vi "Msg.vi"(7 "Actor in":refnum<class "Actor.lvclass">, 11 "Stop Msg in":refnum<class "Stop Msg.lvclass">) -> (0 "Error out":errorcluster, 5 "Actor out":refnum<class "Actor.lvclass">)   [LabVIEW 2025, in "jettl.lvlib" / "Stop Msg.lvlib" / "Stop Msg.lvclass"]
uses:
  Stop Msg.lvclass
  Actor/Actor/Actor.lvclass
  Stop/Stop.lvclass
  Stop Msg.lvclass/Stop Msg.ctl
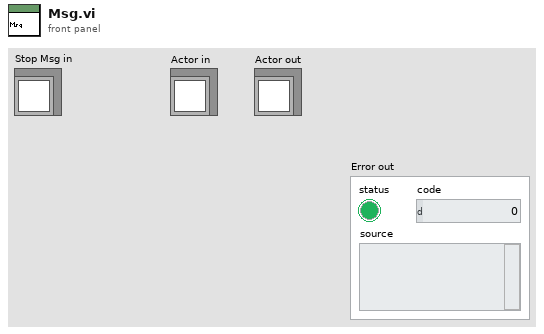
[diagram p1: front panel]
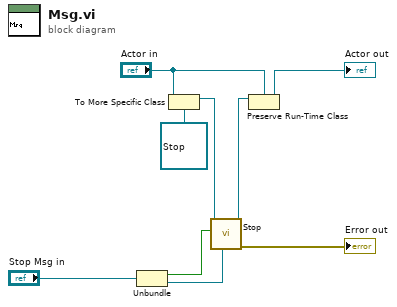
[diagram p0: block diagram]
diagram:
  n1 = Unbundle "Unbundle"("Stop Msg in") -> (w2:bool, w1:refnum<class "Teller.lvclass">)
  n2 = To More Specific Class(target class=refnum<class "Stop.lvclass"> refnum ("Destroy.lvlib:Destroy.lvclass"), reference="Actor in") -> (specific class reference=w5:refnum<class "Stop.lvclass">)  [unwired: 1 in, 1 out]
  n3 = call-dynamic "Stop.vi"("Teller"=w1, "Safe Stop"=w2, "Stop in"=w5) -> ("Error out"=→"Error out":errorcluster, "Stop out"=w4:refnum<class "Stop.lvclass">)  [unwired: 7 in]
  n4 = Preserve Run-Time Class(object in=w4, 2:"Actor in") -> (object out=→"Actor out":refnum<class "Actor.lvclass">)  [unwired: 1 in, 1 out]
